vi "icListen 3 Synchronization.vi"() -> ()   [LabVIEW 2020, in "PAM Library.lvlib"]
uses:
  PAM Library.lvlib
panel:
  out "icListen 3 Synchronization":T1
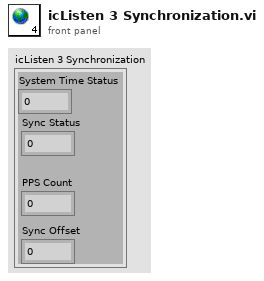
[diagram p1: front panel]
types:
  T1 = cluster{"System Time Status":u8, "Sync Status":u8, "PPS Count":u32, "Sync Offset":u32}
diagram:
